vi "LoggingData.vi"(6 "Start time":u32, 8 "error in":errorcluster, 11 "refnum in":refnum<file>) -> (0 "error out":errorcluster, 3 "refnum out":refnum<file>)   [LabVIEW 2017]
uses:
  Framework/Robot Global Data.vi
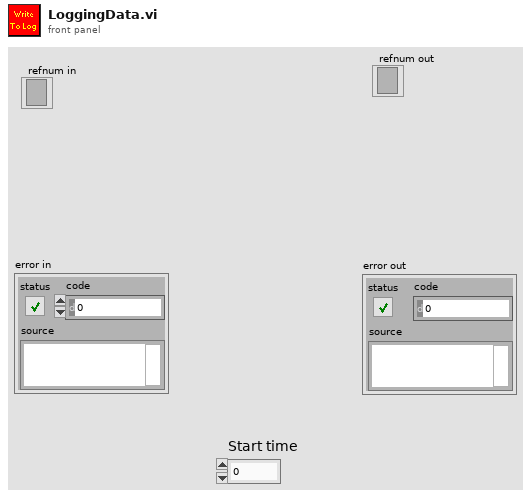
[diagram p1: front panel]
types:
  T1 = typedef "Z900_navX_Flags_OpStatusTypeDef.ctl" = u8
  T2 = typedef "Z900_navX_Flags_CalibrationStatusTypeDef.ctl" = u8
  T3 = cluster{"Update Rate Hz":u8, "Accelerometer Full-Scale Range":u8, "Gyro Full-Scale Range":u16, "OP Status":T1, "Calibration Status":T2, "Sensor Status":cluster{"MOVING":bool, "YAW_STABLE":bool, "MAG_DISTURBANCE":bool, "ALTITUDE_VALID":bool, "SEALEVEL_PRESS_SET":bool, "FUSED_HEADING_VALID":bool}, "Self Test Status":cluster{"Gyro Passed":bool, "Accel Passed":bool, "Mag Passed":bool, "Baro Passed":bool, "Complete":bool}}
  T4 = typedef "WPI_DriverStationRobotMode2.ctl" = enum16{"Autonomous Disabled", "Autonomous Enabled", "Teleop Disabled", "Teleop Enabled", "Disconnected", "Finish", "Test Disabled", "Test Enabled", "Emergency Stopped"}
  T5 = cluster{"MOVING":bool, "YAW_STABLE":bool, "MAG_DISTURBANCE":bool, "ALTITUDE_VALID":bool, "SEALEVEL_PRESS_SET":bool, "FUSED_HEADING_VALID":bool}
  T6 = cluster{"Yaw":dbl, "Roll":dbl, "Pitch":dbl, "Heading":dbl, "Fused Heading":dbl}
  T7 = cluster{"LinearAcceleration X":dbl, "LinearAcceleration Y":dbl, "LinearAcceleration Z":dbl}
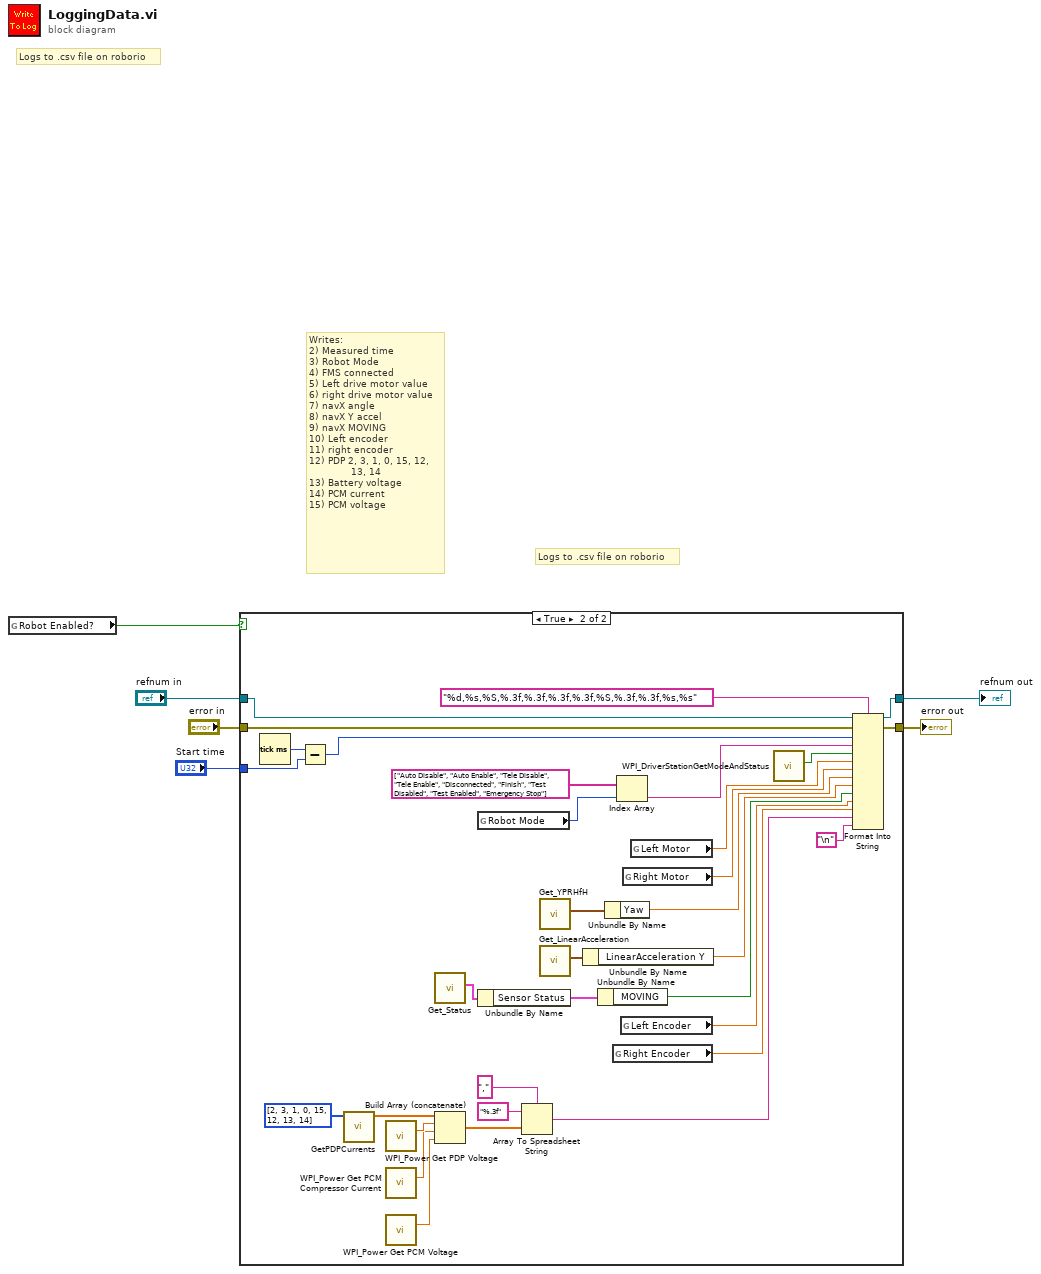
[diagram p0: block diagram]
diagram:
  # "Logs to .csv file on roborio"
  # "Writes:\n2) Measured time\n3) Robot Mode\n4) FMS connected\n5) Left drive motor value\n6) right drive motor value\n7) navX angle\n8) navX Y accel\n9) navX MOVING\n10) Left encoder\n11) right encoder\n12) PDP 2, 3, 1, 0, 15, 12,\n              13, 14\n13) Battery voltage\n14) PCM current\n15) PCM voltage"
  # "Logs to .csv file on roborio"
  n1 = global read "Robot Global Data.vi" "Robot Enabled?"() -> (w1:bool)
  n2 = case shown="True" w1 {
    tunnel: "error in" -> [w7 w41]
    tunnel: "refnum in" -> [w8 w40]
    tunnel: [w8 w39] -> w5
    tunnel: [w7 w38] -> w4
    tunnel: "Start time" -> [_ w37]
    frame False {
    }
    frame True {
      n3 = Tick Count (ms)() -> (millisecond timer value=w31:u32)
      n4 = Subtract(x=w31, y=w37) -> (x-y=w29:u32)
      n5 = call "GetPDPCurrents.vi"("Channels"=i32[] [2, 3, 1, 0, 15, 12, 13, 14]) -> ("Currents"=w23:dbl[])  [unwired: 10 in]
      n6 = call <vilib>:"WPI_Power Get PDP Voltage.vi"() -> ("voltage (V)"=w34:dbl)  [unwired: 14 in, 1 out]
      n7 = call <vilib>:"WPI_Power Get PCM Compressor Current.vi"() -> ("current (A)"=w33:dbl)  [unwired: 14 in, 1 out]
      n8 = call <vilib>:"WPI_Power Get PCM Voltage.vi"() -> ("Input Voltage"=w32:dbl)  [unwired: 13 in, 2 out]
      n9 = call <vilib>:"Get_Status.vi"() -> ("Status"=w18:T3)  [unwired: 11 in]
      n10 = Build Array (concatenate)(w23, w34, w33, w32) -> (w24:dbl[])
      n11 = global read "Robot Global Data.vi" "Robot Mode"() -> (w21:T4)
      n12 = Unbundle By Name(w18) -> ("Sensor Status"=w35:T5)
      n13 = Array To Spreadsheet String(delimiter (Tab)=",", array=w24, 3:"%.3f" ("format string")) -> (spreadsheet string=w10:string)
      n14 = call <vilib>:"Get_YPRHfH.vi"() -> ("YRPHfH"=w20:T6)  [unwired: 11 in]
      n15 = call <vilib>:"Get_LinearAcceleration.vi"() -> ("Linear Acceleration"=w19:T7)  [unwired: 11 in]
      n16 = Unbundle By Name(w19) -> ("LinearAcceleration Y"=w14:dbl)
      n17 = Unbundle By Name(w35) -> ("MOVING"=w13:bool)
      n18 = Unbundle By Name(w20) -> ("Yaw"=w15:dbl)
      n19 = global read "Robot Global Data.vi" "Right Encoder"() -> (w11:dbl)
      n20 = Index Array(array=string[] ["Auto Disable", "Auto Enable", "Tele Disable", "Tele Enable", "Disconnected", "Finish", "Test Disabled", "Test Enabled", "Emergency Stop"], index=w21) -> (element=w28:string)
      n21 = global read "Robot Global Data.vi" "Left Encoder"() -> (w12:dbl)
      n22 = global read "Robot Global Data.vi" "Right Motor"() -> (w16:dbl)
      n23 = global read "Robot Global Data.vi" "Left Motor"() -> (w17:dbl)
      n24 = call <vilib>:"WPI_DriverStationGetModeAndStatus.vi"() -> ("FMS Attached"=w27:bool)  [unwired: 10 in, 1 out]
      n25 = Format Into String(format string="%d,%s,%S,%.3f,%.3f,%.3f,%.3f,%S,%.3f,%.3f,%s,%s", initial string=w40, error in=w41, w29, w28, w27, w17, w16, w15, w14, w13, w12, w11, w10, "\n") -> (resulting string=w39:refnum<file>, error out=w38:errorcluster)
    }
  }
  "refnum out" <- w5
  "error out" <- w4
